vi "Get Maximum Velocity.vi"(4 "error in (no error)":errorcluster, 6 "Axis (1)":i32=1 min=1 max=3, 7 "VISA resource name":refnum<visa-resource-name>) -> (0 "error out":errorcluster, 2 "Maximum Velocity (units/s)":dbl format="%.4g", 3 "VISA resource name out":refnum<visa-resource-name>)   [LabVIEW 2010, in "Newport ESP301.lvlib"]
doc: "Reads the maximum velocity value for an axis."
uses:
  <userlib>/Newport ESP301/Newport ESP301.lvlib
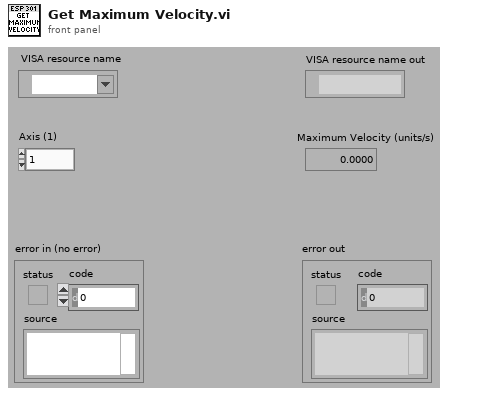
[diagram p1: front panel]
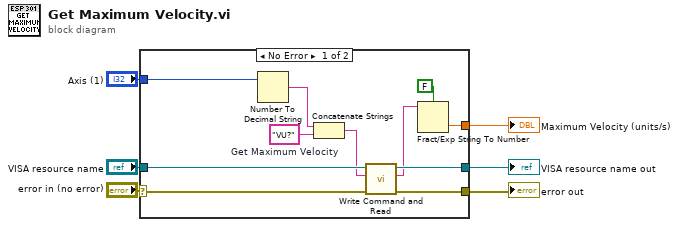
[diagram p0: block diagram]
diagram:
  n1 = case shown="No Error" "error in (no error)" {
    selector: "error in (no error)" -> [w14 w19]
    tunnel: [w16 w19] -> w6
    tunnel: "VISA resource name" -> [w17 w18]
    tunnel: [w15 w18] -> w5
    tunnel: [w12 _] -> w2
    tunnel: "Axis (1)" -> [w9 _]
    frame No Error {
      w11 = "VU?"  # Get Maximum Velocity
      n2 = Number To Decimal String(number=w9) -> (decimal integer string=w10:string)  [unwired: 1 in]
      n3 = Concatenate Strings(w10, w11) -> (w8:string)
      n4 = call <userlib>:"Write Command and Read.vi"("error in (no error)"=w14, "Command"=w8, "VISA resource name"=w17) -> ("error out"=w16:errorcluster, "Returned string"=w13:string, "VISA resource name out"=w15:refnum<visa-resource-name>)  [unwired: 4 in]
      n5 = Fract/Exp String To Number(use system decimal point (T)=FALSE ("utiliser le séparateur décimal du système (V)"), string=w13) -> (number=w12:dbl)  [unwired: 2 in, 1 out]
    }
    frame Error {
    }
  }
  "error out" <- w6
  "VISA resource name out" <- w5
  "Maximum Velocity (units/s)" <- w2
